vi "Test Draw To Picture ARGB.vi"(8 "error in (no error)":errorcluster, 11 "Test Case in":refnum<class "01_Image.lvclass">) -> (0 "error out":errorcluster, 3 "Test Case Out":refnum<class "01_Image.lvclass">)   [LabVIEW 2020, in "test.lvlib" / "01_Image.lvclass"]
uses:
  01_Image.lvclass
  C:/Program Files (x86)/National Instruments/LabVIEW 2026/vi.lib/Astemes/LUnit/Test Case.lvclass
  common/Image Size (Integer).ctl
  image/Image Draw Offset.ctl
  <vilib>/Astemes/LUnit/Test Case.lvclass/Test Case.ctl
  4993e8ee-a06a-463a-9684-69129f64d5ce.vi
  image/New Image.vi
  image/New Image (ARGB Preallocated).vi
  image/Copy Array to Image.vi
  image/Copy Array to Image (ARGB).vi
  image/Draw Image to Picture (ARGB).vi/8cd07b1b-062e-4fe4-9e87-2eb3dc89fe0e.vi
  <vilib>/Astemes/LUnit/Core/LUnit Test Case/Private/Append Pass Result.vi
  <vilib>/Astemes/LUnit/Core/LUnit Test Case/Private/Append Fail Result.vi
  4993e8ee-a06a-463a-9684-69129f64d5ce.vi/9c5d11cd-9439-4240-a1ee-d9baace9c924.vi
  image/New Image (ARGB Preallocated).vi/3321fa97-f432-4e1e-8db9-a0df79aed21b.vi
  image/ARGB Colour to U32 Pixel Value.vi
  <vilib>/Astemes/LUnit/Core/LUnit Test Case/Private/Run In UI.vi
  <vilib>/Utility/error.llb/Clear Errors.vi
  <vilib>/Utility/error.llb/Error Cluster From Error Code.vi
  image/image.lvlib
  common/common.lvlib
panel:
  out "Actual":picture
  out "Expected":picture
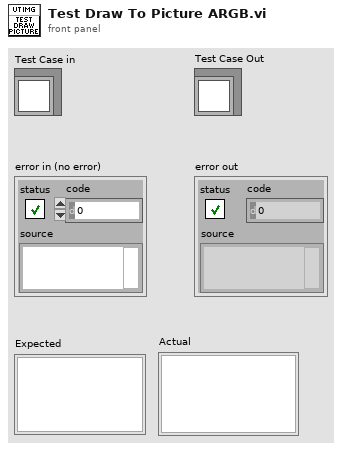
[diagram p1: front panel]
types:
  T1 = typedef "image.lvlib/Image Draw Offset.ctl" = cluster{"Left":i16, "Top":i16}
  T2 = typedef "common.lvlib/Image Size (Integer).ctl" = cluster{"Width":u16, "Height":u16}
  T3 = typedef "image.lvlib/ARGB Image.ctl" = refnum<data-value>
  T4 = typedef "imagedata.ctl" = cluster{"image type":i32, "image depth":i32, "image":u8[], "mask":u8[], "colors":u32[], "Rectangle":cluster{"left":i16, "top":i16, "right":i16, "bottom":i16}}
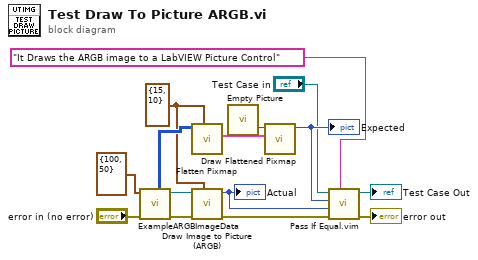
[diagram p0: block diagram]
diagram:
  w1 = T1 {"Left"=15, "Top"=10} ("Image Draw Offset (Default 0,0)")
  n1 = call "ExampleARGBImageData.vi"("error in (no error)"="error in (no error)", "Image Size"=T2 {"Width"=100, "Height"=50} ("Preallocated Image Size (Default - 0,0)")) -> ("error out"=w4:errorcluster, "Data Value Reference out"=w3:T3, "ARGB Array Data"=w2:u32[][])  [unwired: 6 in, 1 out]
  n2 = call <vilib>:"Flatten Pixmap.vi"("top left"=w1, "24-bit pixmap"=w2) -> ("image data"=w10:T4)  [unwired: 9 in]
  n3 = call "Draw Image to Picture (ARGB).vi"("Image Draw Offset (Default 0,0)"=w1, "error in (no error)"=w4, "ARGB Image Source in"=w3) -> ("error out"=w11:errorcluster, "Picture"=w7:picture)  [unwired: 7 in]
  "Actual" <- w7
  n4 = call "Empty Picture"() -> ("empty picture"=w9:picture)
  n5 = call <vilib>:"Draw Flattened Pixmap.vi"("image data"=w10, "picture"=w9) -> ("new picture"=w8:picture)  [unwired: 7 in]
  "Expected" <- w8
  n6 = call "Pass If Equal.vim"("Description"="It Draws the ARGB image to a LabVIEW Picture Control", "error in (no error)"=w11, "Actual"=w7, "Expected"=w8, "LUnit Test Case In"="Test Case in") -> ("error out"=→"error out":errorcluster, "LUnit Test Case Out"=→"Test Case Out":refnum<class "01_Image.lvclass">)  [unwired: 5 in]
